vi "Save config.vi"(8 "error in (no error)":errorcluster, 11 "Datos Adquisición":T1={"Equipo a Utilizar"=enum."TDS 2012B Osciloscope", "Montura"=enum."Motor Bipolar", "Datos Zaber"={"Sentido de Adquisición"=FALSE, "Comenzar Desde Home?"=FALSE, "Distancia a recorrer (um)"=0.0, "Pasos motor"=0, "Distancia entre Lecturas (um)"=0.0, "Puerto"=""}, "Datos Bipolar/Unipolar"={"Puerto COM"="", "Pasos entre Lecturas"=0, "Numero de lecturas"=0, "Sentido del motor"=TRUE}, "Datos Archivo"={"Ruta Archivo"=path "", "Nombre de Prueba"=""}, "Datos actuales"={"Montura"="", "Equipo"="", "Posición Actual"="", "Distancia Total a recorrer"="", "distancia Entre lecturas"="", "Pasos entre lecturas"=""}, "Datos a Guardar In"={"Datos Cursor Tektronix"="", "Datos Lokin"="", "Posición Cero"=0.0, "Posición Actual"=0.0}, "Datos Osciloscopio"={"Sesión Visa Osciloscopio"="Tektronix_TDS2012C", "Tipo de Adquisición"=enum."Voltaje Pico Pico", "Canal a Utilizar"=enum."Canal 1", "Parametros de Adquisición"=enum."Una Muestra", "Número Promedio"=2}, "Datos Lock In"={"Visa Lock in"="Tektronix_TDS2012C"}} {"Datos Osciloscopio"."Número Promedio" min=2 max=20; "Datos a Guardar In"."Posición Actual" format="%#_10f"; "Datos a Guardar In"."Posición Cero" format="%#_10f"; "Datos Bipolar/Unipolar"."Numero de lecturas" max=910098 step=1}) -> (0 "error out":errorcluster)   [LabVIEW 2020]
uses:
  <vilib>/Utility/config.llb/NI_LVConfig.lvlib
  <vilib>/Utility/config.llb/Write Key (I32).vi
  Type Definitions/Datos Zaber.ctl
  Type Definitions/parametros motores.ctl
  Type Definitions/Datos a Guardar.ctl
  Type Definitions/datos osciloscopio.ctl
  H:/Mi unidad/Departamento de Ingenieria/Investigadores/Gabriel Ramos/Proyecto Monturas v13/LV Source/Type Definitions/Tipos de montura.ctl
  Type Definitions/Asistente de adquisicion Cluster.ctl
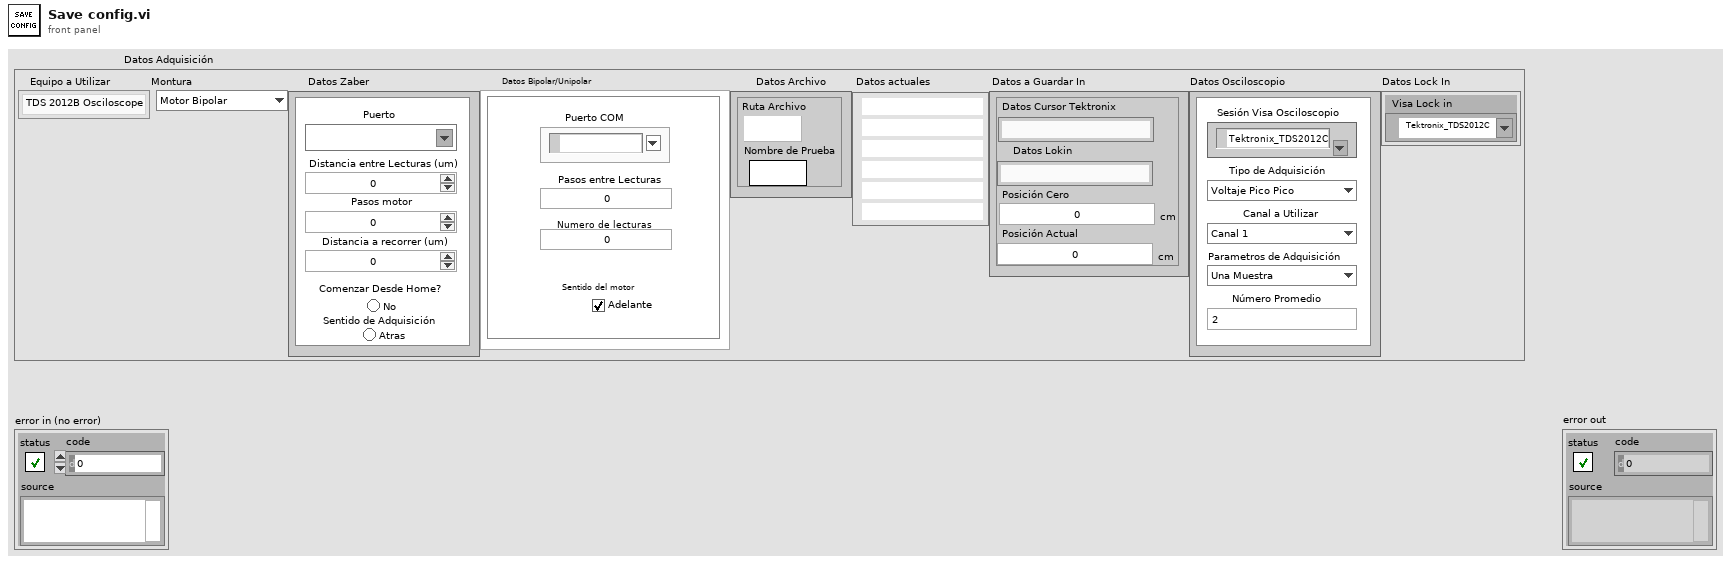
[diagram p1: front panel]
types:
  T1 = typedef "Asistente de adquisicion Cluster.ctl" = cluster{"Equipo a Utilizar":enum16{"SR830 Lock In", "TDS 2012B Osciloscope"}, "Montura":T2, "Datos Zaber":T3, "Datos Bipolar/Unipolar":T4, "Datos Archivo":cluster{"Ruta Archivo":path, "Nombre de Prueba":string}, "Datos actuales":cluster{"Montura":string, "Equipo":string, "Posición Actual":string, "Distancia Total a recorrer":string, "distancia Entre lecturas":string, "Pasos entre lecturas":string}, "Datos a Guardar In":T5, "Datos Osciloscopio":T6, "Datos Lock In":cluster{"Visa Lock in":refnum<visa-resource-name>}}
  T2 = typedef "Tipos de montura.ctl" = enum16{"Zaber T-LSR450B", "Zaber-T-LSR300B", "Zaber-T-LSRxxx", "Motor Bipolar", "Motor Unipolar"}
  T3 = typedef "Datos Zaber.ctl" = cluster{"Sentido de Adquisición":bool, "Comenzar Desde Home?":bool, "Distancia a recorrer (um)":dbl, "Pasos motor":i32, "Distancia entre Lecturas (um)":dbl, "Puerto":refnum<visa-resource-name>}
  T4 = typedef "parametros motores.ctl" = cluster{"Puerto COM":refnum<visa-resource-name>, "Pasos entre Lecturas":u16, "Numero de lecturas":u32, "Sentido del motor":bool}
  T5 = typedef "Datos a Guardar.ctl" = cluster{"Datos Cursor Tektronix":string, "Datos Lokin":string, "Posición Cero":dbl[unit], "Posición Actual":dbl[unit]}
  T6 = typedef "datos osciloscopio.ctl" = cluster{"Sesión Visa Osciloscopio":refnum<visa-resource-name>, "Tipo de Adquisición":enum16{"Voltaje Pico Pico", "Voltaje RMS", "Cursor Tiempo"}, "Canal a Utilizar":enum16{"Canal 1", "Canal 2", "Canal 1 y 2"}, "Parametros de Adquisición":enum16{"Una Muestra", "Promedio"}, "Número Promedio":i32}
  T7 = cluster{"Visa Lock in":refnum<visa-resource-name>}
  T8 = typedef "NI_LVConfig.lvlib/Config Data RefNum.ctl" = refnum<k1>
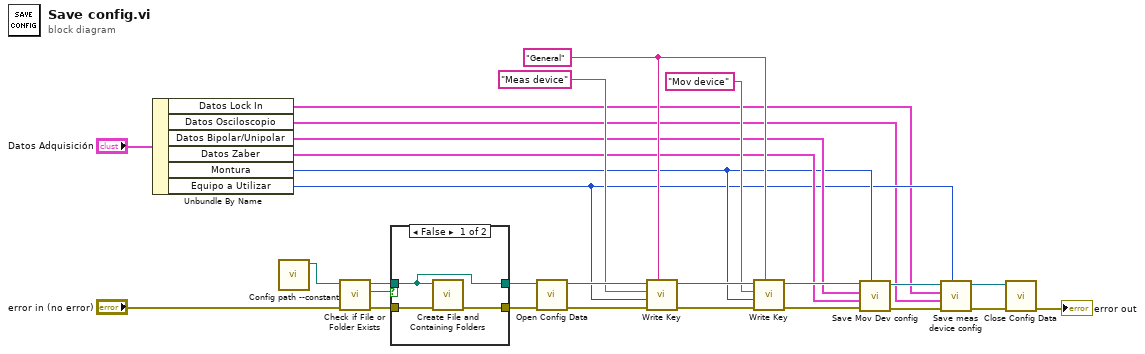
[diagram p0: block diagram]
diagram:
  w14 = "General"
  n1 = Unbundle By Name("Datos Adquisición") -> ("Datos Lock In"=w1:T7, "Datos Osciloscopio"=w2:T6, "Datos Bipolar/Unipolar"=w9:T4, "Datos Zaber"=w10:T3, "Montura"=w8:T2, "Equipo a Utilizar"=w3:enum16{"SR830 Lock In", "TDS 2012B Osciloscope"})
  n2 = call "Config path --constant.vi"() -> ("appended path"=w28:path)  [unwired: 11 in]
  n3 = call <vilib>:"Check if File or Folder Exists.vi"("error in (no error)"="error in (no error)", "path"=w28) -> ("error out"=w23:errorcluster, "file or folder exists?"=w26:bool, "dup path"=w25:path)  [unwired: 7 in]
  n4 = case shown="False" w26 {
    tunnel: w25 -> [w29 w33]
    tunnel: [w29 w33] -> w24
    tunnel: w23 -> [w31 w32]
    tunnel: [w30 w32] -> w22
    frame False {
      n5 = call <vilib>:"Create File and Containing Folders.vi"("error in (no error)"=w31, "file path"=w29) -> ("error out"=w30:errorcluster)  [unwired: 8 in, 1 out]
    }
    frame True {
    }
  }
  n6 = call <vilib>:"Open Config Data.vi"("error in (no error)"=w22, "configuration file path"=w24) -> ("error out"=w21:errorcluster, "refnum"=w17:T8)  [unwired: 7 in, 1 out]
  n7 = call-poly <vilib>:"Write Key.vi"("section"=w14, "error in (no error)"=w21, "value"=w3, "key"="Meas device", "refnum"=w17) -> ("error out"=w18:errorcluster, "refnum out"=w15:T8)  [unwired: 4 in, 1 out]
  n8 = call-poly <vilib>:"Write Key.vi"("section"=w14, "error in (no error)"=w18, "value"=w8, "key"="Mov device", "refnum"=w15) -> ("error out"=w11:errorcluster, "refnum out"=w12:T8)  [unwired: 4 in, 1 out]
  n9 = call "Save Mov Dev config.vi"("Montura"=w8, "error in (no error)"=w11, "Datos Zaber"=w10, "Datos Bipolar/Unipolar"=w9, "Refnum in"=w12) -> ("error out"=w7:errorcluster, "refnum out"=w5:T8)  [unwired: 5 in]
  n10 = call "Save meas device config.vi"("Equipo a Utilizar"=w3, "error in (no error)"=w7, "Datos Osciloscopio"=w2, "Datos Lock In"=w1, "Refnum in"=w5) -> ("error out"=w6:errorcluster, "Refnum out"=w4:T8)  [unwired: 5 in]
  n11 = call <vilib>:"Close Config Data.vi"("error in (no error)"=w6, "refnum"=w4) -> ("error out"=→"error out":errorcluster)  [unwired: 8 in, 1 out]
